vi "version_2_2_GUI.vi"() -> ()   [LabVIEW 2019]
uses:
  <vilib>/Native 3D Graph/xcontrol/3DPC_SurfacePlot.xctl
  <vilib>/DAQmx/write.llb/DAQmx Write (Digital Bool 1Line 1Point).vi
  <vilib>/DAQmx/create/channels.llb/DAQmx Create Channel (DO-Digital Output).vi
  <vilib>/DAQmx/miscellaneous.llb/DAQmx Fill In Error Info.vi
  <vilib>/DAQmx/create/channels.llb/DAQmx Create Channel (CO-Pulse Generation-Frequency).vi
  <vilib>/DAQmx/configure/timing.llb/DAQmx Timing (Implicit).vi
  <vilib>/Utility/file.llb/Read Delimited Spreadsheet (DBL).vi
  <resource>/objmgr/daqmx.rc
panel:
  in  "Stop Scanning":bool
  in  "3D View":refnum<k7>(container)
  in  "Step Signal X":tag
  in  "Direction x":tag
  in  "Enable  X":tag
  in  "Direction Y":tag
  in  "Enable Y  2":tag
  in  "Step Signal Y":tag
  in  "dir?":bool
  in  "Dir? 2":bool
  in  "Enable Y":bool
  in  "Enable X":bool
  in  "stop 2":bool
  in  "data pass":bool
  in  "Data file":path
  out "Y  mm":dbl
  in  "X distance mm":dbl
  out "X mm":dbl
  in  "Stop chart":bool
  out "Hieght":dbl
  out "Amplitude Chart":dynamicdata(graph)
  out "3D Graph":refnum<class "Base Datatype.lvclass">[](xcontrol)
  # "xy stage connection"
  # "@Blueacre Technology"
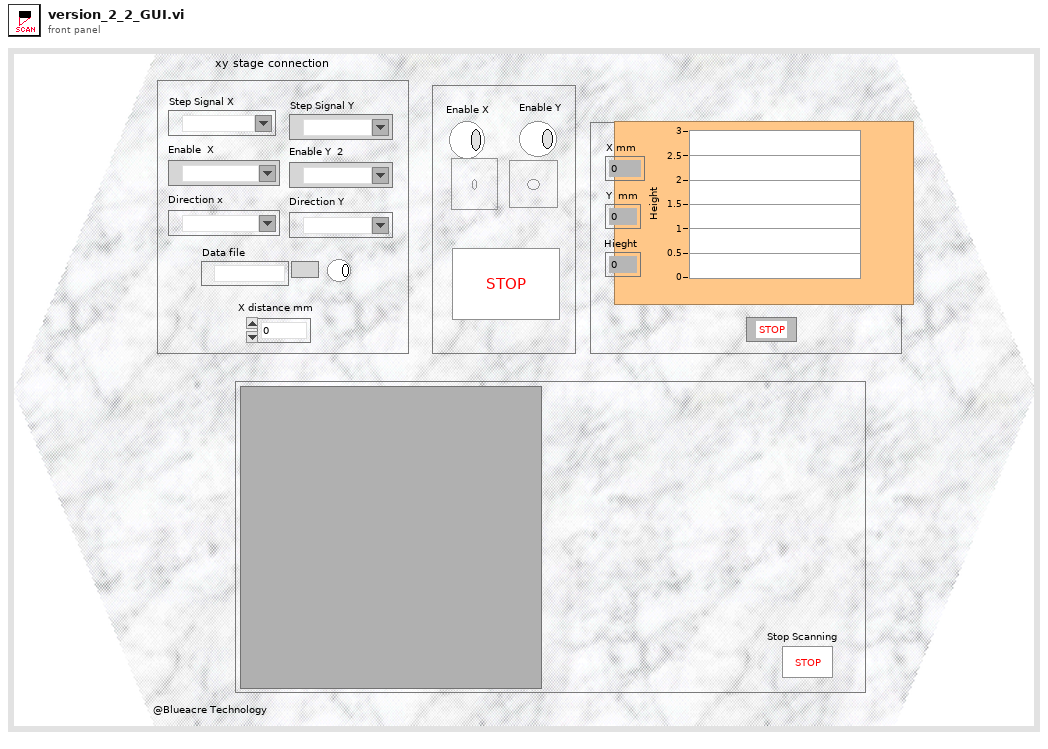
[diagram p1: front panel]
types:
  T1 = enum16{"open", "replace", "create", "open or create", "replace or create", "replace or create with confirmation"}
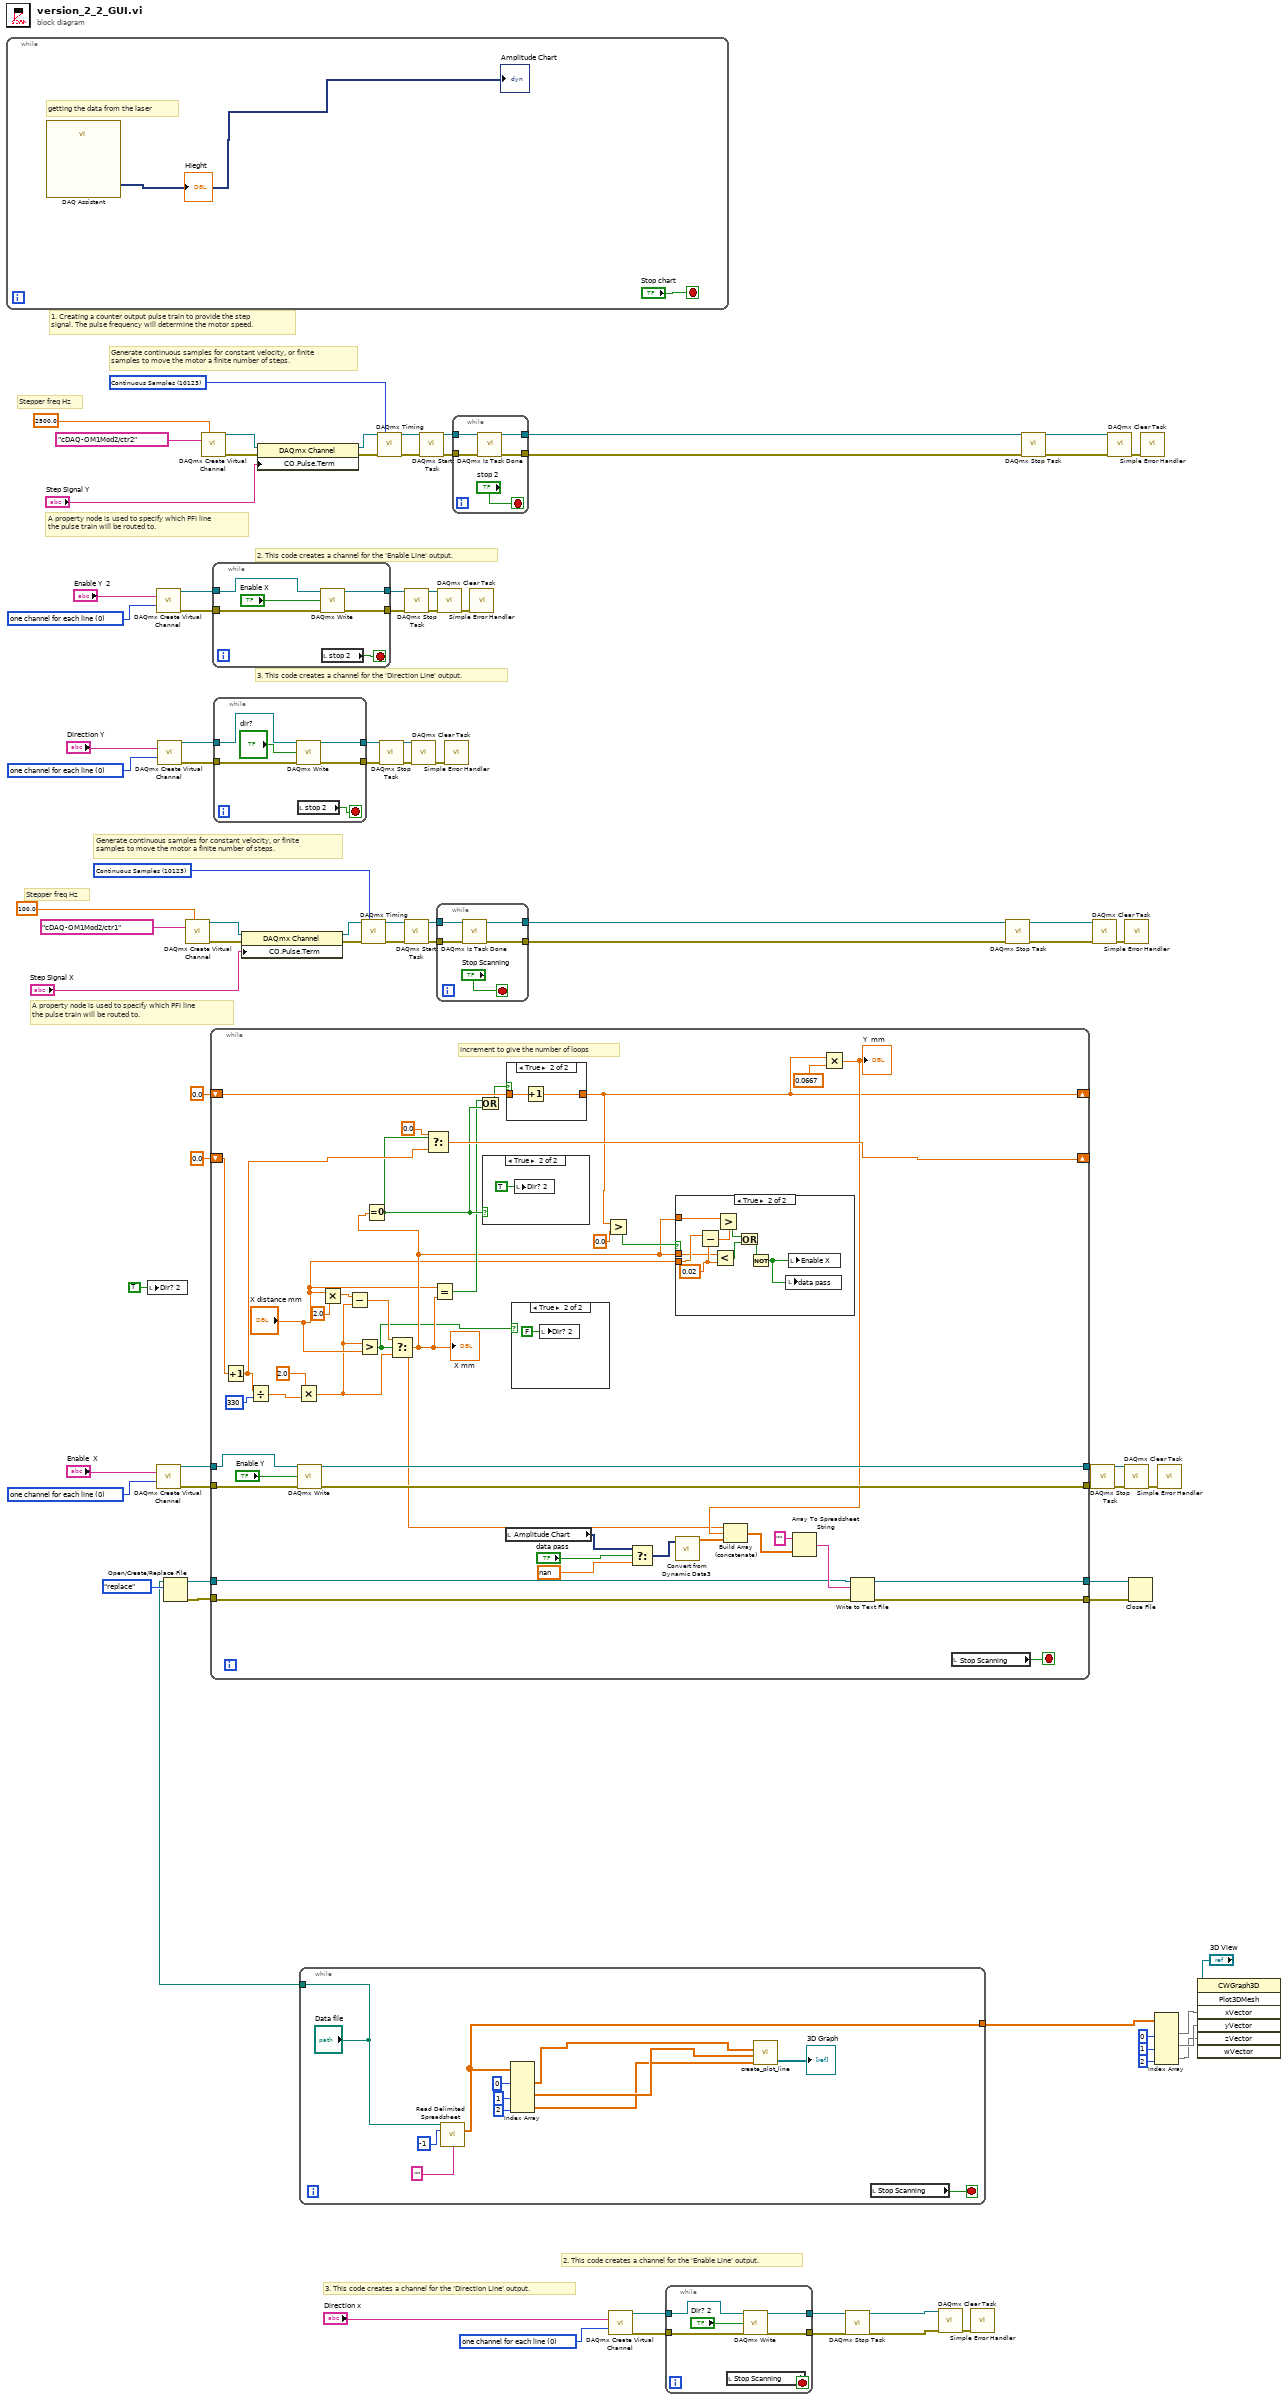
[diagram p0: block diagram]
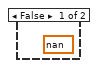
[diagram p4: hidden frame]
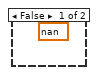
[diagram p5: hidden frame]
diagram:
  w20 = 10123 items=["Finite Samples"=10178, "Continuous Samples"=10123, "Hardware Timed Single Point"=12522] ("sample mode")
  w37 = 0 items=["one channel for each line", "one channel for all lines"] ("line grouping")
  w52 = 0 items=["one channel for each line", "one channel for all lines"] ("line grouping")
  w56 = 0 items=["one channel for each line", "one channel for all lines"] ("line grouping")
  w71 = 0 items=["one channel for each line", "one channel for all lines"] ("line grouping")
  w87 = 10123 items=["Finite Samples"=10178, "Continuous Samples"=10123, "Hardware Timed Single Point"=12522] ("sample mode")
  # "Stepper freq Hz"
  # "Stepper freq Hz"
  # "Generate continuous samples for constant velocity, or finite \nsamples to move the motor a finite number of steps."
  # "A property node is used to specify which PFI line \nthe pulse train will be routed to."
  # "3. This code creates a channel for the 'Direction Line' output."
  # "2. This code creates a channel for the 'Enable Line' output."
  # "Generate continuous samples for constant velocity, or finite \nsamples to move the motor a finite number of steps."
  # "A property node is used to specify which PFI line \nthe pulse train will be routed to."
  # "3. This code creates a channel for the 'Direction Line' output."
  # "2. This code creates a channel for the 'Enable Line' output."
  # "1. Creating a counter output pulse train to provide the step\nsignal. The pulse frequency will determine the motor speed."
  n1 = while {
    stop <- "Stop chart" stop-if-true
    # "getting the data from the laser"
    n2 = call "DAQ Assistant"() -> ("data"=→"Hieght" →"Amplitude Chart":dynamicdata)  [unwired: 16 in, 3 out]
  }
  n3 = local write "Dir? 2"(TRUE ("Dir? 2")) -> ()
  n4 = call-poly <vilib>:"DAQmx Create Virtual Channel.vi"("lines"="Enable Y  2", "line grouping"=w71) -> ("task out"=w70:refnum<k21>, "error out"=w69:errorcluster)  [unwired: 12 in]
  n5 = call-poly <vilib>:"DAQmx Create Virtual Channel.vi"("lines"="Enable  X", "line grouping"=w52) -> ("task out"=w51:refnum<k21>, "error out"=w50:errorcluster)  [unwired: 12 in]
  n6 = call-poly <vilib>:"DAQmx Create Virtual Channel.vi"("lines"="Direction Y", "line grouping"=w56) -> ("task out"=w57:refnum<k21>, "error out"=w58:errorcluster)  [unwired: 12 in]
  n7 = call-poly <vilib>:"DAQmx Create Virtual Channel.vi"("frequency"=100.0, "counter"=tag "cDAQ-OM1Mod2/ctr1") -> ("task out"=w30:refnum<k21>, "error out"=w31:errorcluster)  [unwired: 12 in]
  n8 = call-poly <vilib>:"DAQmx Create Virtual Channel.vi"("frequency"=2500.0, "counter"=tag "cDAQ-OM1Mod2/ctr2") -> ("task out"=w77:refnum<k21>, "error out"=w76:errorcluster)  [unwired: 12 in]
  n9 = while {
    tunnel: w70 -> [w95]
    tunnel: w69 -> [w94]
    tunnel: [w93] -> w68
    tunnel: [w92] -> w67
    stop <- w90 stop-if-true
    n10 = call-poly <vilib>:"DAQmx Write.vi"("task/channels in"=w95, "data"="Enable X", "error in"=w94) -> ("task out"=w93:refnum<k21>, "error out"=w92:errorcluster)  [unwired: 10 in, 1 out]
    n11 = local read "stop 2"() -> (w90:bool)
  }
  n12 = while {
    tunnel: w57 -> [w101]
    tunnel: w58 -> [w100]
    tunnel: [w99] -> w59
    tunnel: [w98] -> w60
    stop <- w96 stop-if-true
    n13 = call-poly <vilib>:"DAQmx Write.vi"("task/channels in"=w101, "data"="dir?", "error in"=w100) -> ("task out"=w99:refnum<k21>, "error out"=w98:errorcluster)  [unwired: 10 in, 1 out]
    n14 = local read "stop 2"() -> (w96:bool)
  }
  n15 = property class="DAQmx Channel"(reference=w30, error in=w31, "CO.Pulse.Term"="Step Signal X") -> (reference out=w32:refnum<k21>, error out=w33:errorcluster)
  n16 = property class="DAQmx Channel"(reference=w77, error in=w76, "CO.Pulse.Term"="Step Signal Y") -> (reference out=w75:refnum<k21>, error out=w74:errorcluster)
  n17 = while {
    tunnel: [w111] -> w2
    tunnel: ["Data file"] -> w1
    stop <- w104 stop-if-true
    n18 = call-poly <vilib>:"Read Delimited Spreadsheet.vi"("file path (dialog if empty)"="Data file", "number of rows (all:-1)"=-1, "delimiter (\\t)"="" ("delimiter (\\t)")) -> ("all rows"=w111:dbl[][])  [unwired: 7 in, 5 out]
    n19 = Index Array(array=w111, index (col) #1=0 ("disabled index (col)"), index (col) #2=1 ("disabled index (col)"), index (col) #3=2 ("index (col)")) -> (element #1=w112:dbl[], element #2=w113:dbl[], element #3=w110:dbl[])  [unwired: 3 in]
    n20 = call <vilib>:"create_plot_line.vi"("z vector"=w110, "y vector"=w113, "x vector"=w112) -> ("plots out"=→"3D Graph":refnum<class "Base Datatype.lvclass">[])  [unwired: 2 in, 6 out]
    n21 = local read "Stop Scanning"() -> (w104:bool)
  }
  n22 = Open/Create/Replace File(file path (use dialog)=w1, operation (0:open)=T1."replace") -> (refnum out=w13:refnum<file>, error out=w14:errorcluster)  [unwired: 4 in, 1 out]
  n23 = while {
    tunnel: w51 -> [w154]
    tunnel: w50 -> [w153]
    tunnel: [w152] -> w49
    tunnel: [w151] -> w48
    shift-right: [w145] -> _
    shift-left: 0.0 -> [w142]
    shift-right: [w122] -> _
    shift-left: 0.0 -> [w138]
    tunnel: w14 -> [w132]
    tunnel: w13 -> [w131]
    tunnel: [w130] -> w12
    tunnel: [w129] -> w11
    stop <- w150 stop-if-true
    # "increment to give the number of loops"
    n24 = Increment(x=w142) -> (x+1=w141:dbl)
    n25 = Divide(x=w141, y=330) -> (x/y=w146:dbl)
    n26 = Multiply(x=2.0, y=w146) -> (x*y=w119:dbl)
    n27 = call-poly <vilib>:"DAQmx Write.vi"("task/channels in"=w154, "data"="Enable Y", "error in"=w153) -> ("task out"=w152:refnum<k21>, "error out"=w151:errorcluster)  [unwired: 10 in, 1 out]
    n28 = Multiply(x="X distance mm", y=2.0) -> (x*y=w140:dbl)
    n29 = Subtract(x=w140, y=w119) -> (x-y=w143:dbl)
    n30 = Greater?(x=w119, y="X distance mm") -> (0:w118:bool)
    n31 = Select(t=w143, s=w118, f=w119) -> (s? t:f=w121:dbl)
    "X mm" <- w121
    n32 = Equal To 0?(x=w121) -> (x = 0?=w125:bool)
    n33 = Select(t=0.0, s=w125, f=w141) -> (s? t:f=w145:dbl)
    n34 = Equal?(x="X distance mm", y=w121) -> (x = y?=w124:bool)
    n35 = Or(x=w124, y=w125) -> (x .or. y?=w123:bool)
    n36 = case shown="True" w125 {
      frame False {
        (unwired) nan
      }
      frame True {
        n37 = local write "Dir? 2"(TRUE ("Dir? 2")) -> ()
      }
    }
    n38 = local read "Amplitude Chart"() -> (w117:dynamicdata)
    n39 = case shown="True" w123 {
      tunnel: w138 -> [w164 w166]
      tunnel: [w164 w165] -> w122
      frame False {
      }
      frame True {
        n40 = Increment(x=w166) -> (x+1=w165:dbl)
      }
    }
    n41 = case shown="True" w118 {
      frame False {
        (unwired) nan
      }
      frame True {
        n42 = local write "Dir? 2"(FALSE ("Dir? 2")) -> ()
      }
    }
    n43 = Greater?(x=w122, y=0.0) -> (0:w137:bool)
    n44 = Select(t=w117, s="data pass", f=nan) -> (s? t:f=w115:dynamicdata)
    n45 = case shown="True" w137 {
      tunnel: w121 -> [_ w161]
      tunnel: "X distance mm" -> [_ w162]
      tunnel: w121 -> [_ w156]
      frame False {
      }
      frame True {
        w163 = 0.02 ("y")
        n46 = Subtract(x=w162, y=w163) -> (x-y=w160:dbl)
        n47 = Less?(x=w161, y=w163) -> (x < y?=w158:bool)
        n48 = Greater?(x=w156, y=w160) -> (0:w159:bool)
        n49 = Or(x=w159, y=w158) -> (x .or. y?=w157:bool)
        n50 = Not(x=w157) -> (.not. x?=w155:bool)
        n51 = local write "data pass"(w155) -> ()
        n52 = local write "Enable X"(w155) -> ()
      }
    }
    n53 = call "Convert from Dynamic Data3"("Dynamic Data Type"=w115) -> ("Array"=w127:dbl[])  [unwired: 3 in]
    n54 = Multiply(x=w122, y=0.0667) -> (x*y=w126:dbl)
    "Y  mm" <- w126
    n55 = Build Array (concatenate)(w121, w126, w127) -> (w128:dbl[])
    n56 = Array To Spreadsheet String(array=w128, 3:"" ("format string")) -> (spreadsheet string=w134:string)  [unwired: 1 in]
    n57 = Write to Text File(file (use dialog)=w131, text=w134, error in=w132) -> (refnum out=w129:refnum<file>, error out=w130:errorcluster)  [unwired: 1 in, 1 out]
    n58 = local read "Stop Scanning"() -> (w150:bool)
  }
  n59 = call-poly <vilib>:"DAQmx Timing.vi"("task/channels in"=w32, "sample mode"=w20, "error in"=w33) -> ("task out"=w21:refnum<k21>, "error out"=w22:errorcluster)  [unwired: 11 in]
  n60 = call-poly <vilib>:"DAQmx Timing.vi"("task/channels in"=w75, "sample mode"=w87, "error in"=w74) -> ("task out"=w86:refnum<k21>, "error out"=w85:errorcluster)  [unwired: 11 in]
  n61 = call <vilib>:"DAQmx Stop Task.vi"("task/channels in"=w59, "error in"=w60) -> ("task out"=w61:refnum<k21>, "error out"=w62:errorcluster)  [unwired: 12 in]
  n62 = call <vilib>:"DAQmx Start Task.vi"("task/channels in"=w21, "error in"=w22) -> ("task out"=w23:refnum<k21>, "error out"=w24:errorcluster)  [unwired: 12 in]
  n63 = call <vilib>:"DAQmx Stop Task.vi"("task/channels in"=w68, "error in"=w67) -> ("task out"=w66:refnum<k21>, "error out"=w65:errorcluster)  [unwired: 12 in]
  n64 = call <vilib>:"DAQmx Clear Task.vi"("task in"=w61, "error in"=w62) -> ("error out"=w63:errorcluster)  [unwired: 13 in]
  n65 = call <vilib>:"DAQmx Start Task.vi"("task/channels in"=w86, "error in"=w85) -> ("task out"=w84:refnum<k21>, "error out"=w83:errorcluster)  [unwired: 12 in]
  n66 = while {
    tunnel: w23 -> [w173]
    tunnel: w24 -> [w172]
    tunnel: [w171] -> w25
    tunnel: [w170] -> w26
    stop <- "Stop Scanning" stop-if-true
    n67 = call <vilib>:"DAQmx Is Task Done.vi"("task/channels in"=w173, "error in"=w172) -> ("task out"=w171:refnum<k21>, "error out"=w170:errorcluster)  [unwired: 11 in, 1 out]
  }
  n68 = call <vilib>:"DAQmx Clear Task.vi"("task in"=w66, "error in"=w65) -> ("error out"=w64:errorcluster)  [unwired: 13 in]
  n69 = call <vilib>:"Simple Error Handler.vi"("error in (no error)"=w63) -> ()  [unwired: 4 in, 5 out]
  n70 = while {
    tunnel: w84 -> [w178]
    tunnel: w83 -> [w177]
    tunnel: [w176] -> w82
    tunnel: [w175] -> w81
    stop <- "stop 2" stop-if-true
    n71 = call <vilib>:"DAQmx Is Task Done.vi"("task/channels in"=w178, "error in"=w177) -> ("task out"=w176:refnum<k21>, "error out"=w175:errorcluster)  [unwired: 11 in, 1 out]
  }
  n72 = call <vilib>:"Simple Error Handler.vi"("error in (no error)"=w64) -> ()  [unwired: 4 in, 5 out]
  n73 = call-poly <vilib>:"DAQmx Create Virtual Channel.vi"("lines"="Direction x", "line grouping"=w37) -> ("task out"=w38:refnum<k21>, "error out"=w39:errorcluster)  [unwired: 12 in]
  n74 = while {
    tunnel: w38 -> [w184]
    tunnel: w39 -> [w183]
    tunnel: [w182] -> w40
    tunnel: [w181] -> w41
    stop <- w180 stop-if-true
    n75 = local read "Stop Scanning"() -> (w180:bool)
    n76 = call-poly <vilib>:"DAQmx Write.vi"("task/channels in"=w184, "data"="Dir? 2", "error in"=w183) -> ("task out"=w182:refnum<k21>, "error out"=w181:errorcluster)  [unwired: 10 in, 1 out]
  }
  n77 = call <vilib>:"DAQmx Stop Task.vi"("task/channels in"=w40, "error in"=w41) -> ("task out"=w42:refnum<k21>, "error out"=w43:errorcluster)  [unwired: 12 in]
  n78 = call <vilib>:"DAQmx Clear Task.vi"("task in"=w42, "error in"=w43) -> ("error out"=w44:errorcluster)  [unwired: 13 in]
  n79 = call <vilib>:"Simple Error Handler.vi"("error in (no error)"=w44) -> ()  [unwired: 4 in, 5 out]
  n80 = call <vilib>:"DAQmx Stop Task.vi"("task/channels in"=w25, "error in"=w26) -> ("task out"=w27:refnum<k21>, "error out"=w28:errorcluster)  [unwired: 12 in]
  n81 = call <vilib>:"DAQmx Stop Task.vi"("task/channels in"=w82, "error in"=w81) -> ("task out"=w80:refnum<k21>, "error out"=w79:errorcluster)  [unwired: 12 in]
  n82 = call <vilib>:"DAQmx Stop Task.vi"("task/channels in"=w49, "error in"=w48) -> ("task out"=w47:refnum<k21>, "error out"=w46:errorcluster)  [unwired: 12 in]
  n83 = call <vilib>:"DAQmx Clear Task.vi"("task in"=w27, "error in"=w28) -> ("error out"=w29:errorcluster)  [unwired: 13 in]
  n84 = call <vilib>:"DAQmx Clear Task.vi"("task in"=w80, "error in"=w79) -> ("error out"=w78:errorcluster)  [unwired: 13 in]
  n85 = call <vilib>:"DAQmx Clear Task.vi"("task in"=w47, "error in"=w46) -> ("error out"=w45:errorcluster)  [unwired: 13 in]
  n86 = call <vilib>:"Simple Error Handler.vi"("error in (no error)"=w29) -> ()  [unwired: 4 in, 5 out]
  n87 = Close File(refnum=w11, error in=w12) -> ()  [unwired: 2 out]
  n88 = call <vilib>:"Simple Error Handler.vi"("error in (no error)"=w78) -> ()  [unwired: 4 in, 5 out]
  n89 = Index Array(array=w2, index (col) #1=0 ("disabled index (col)"), index (col) #2=1 ("index (col)"), index (col) #3=2 ("index (col)")) -> (element #1=w6:dbl[], element #2=w5:dbl[], element #3=w4:dbl[])  [unwired: 3 in]
  n90 = call <vilib>:"Simple Error Handler.vi"("error in (no error)"=w45) -> ()  [unwired: 4 in, 5 out]
  n91 = invoke class="CWGraph3D" method="Plot3DMesh"(reference="3D View", "xVector"=w6, "yVector"=w5, "zVector"=w4) -> ()  [unwired: 3 in, 7 out]
